vi "Session Reservation Keys.vi"() -> (3 "session reservation keys":string[](array[string]))   [LabVIEW 2021, in "NI Session Management V1 Client.lvlib" / "Session Reservation.lvclass"]
uses:
  Session Reservation.lvclass
  Session Reservation.lvclass/Session Reservation.ctl
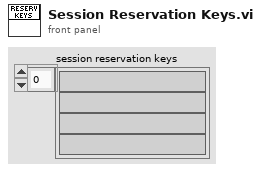
[diagram p1: front panel]
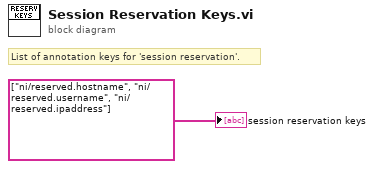
[diagram p0: block diagram]
diagram:
  # "List of annotation keys for 'session reservation'."
  "session reservation keys" <- string[] ["ni/reserved.hostname", "ni/reserved.username", "ni/reserved.ipaddress"] ("reserve annotation keys")
